vi "BufferWork.vi"(8 "SizeOfArray":i32, 11 "InputArray":i32[](array[numeric])) -> (0 "Index":i32, 3 "OutputArray":i32[](array[numeric]))   [LabVIEW 2020]
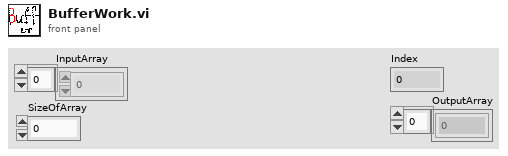
[diagram p1: front panel]
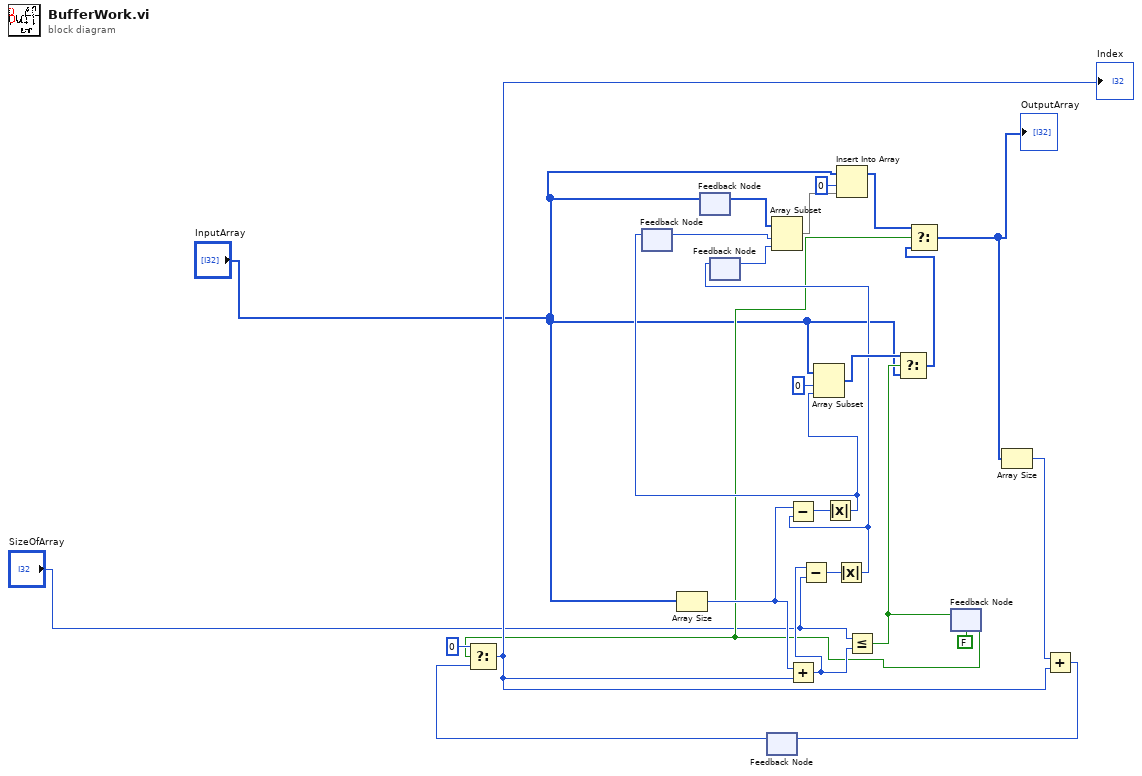
[diagram p0: block diagram]
diagram:
  n1 = feedback #1() -> (w14:i32)  [unwired: 1 in]
  n2 = Array Size(array="InputArray") -> (size(s)=w8:i32)
  n3 = feedback #2() -> (w15:i32[])  [unwired: 1 in]
  n4 = feedback-in #2("InputArray") -> ()
  n5 = feedback #3() -> (w12:i32)  [unwired: 1 in]
  n6 = feedback #4() -> (w4:i32)  [unwired: 1 in]
  n7 = Array Subset(array=w15, index=w14, length=w12) -> (w22:i32[])
  n8 = Insert Into Array(array="InputArray", index=0, new element=w22) -> (w20:i32[])
  n9 = feedback #5(FALSE) -> (w3:bool)
  n10 = Select(t=0, s=w3, f=w4) -> (s? t:f=w6:i32)
  "Index" <- w6
  n11 = Add(x=w8, y=w6) -> (x+y=w9:i32)
  n12 = Subtract(x=w9, y="SizeOfArray") -> (x-y=w16:i32)
  n13 = Absolute Value(x=w16) -> (abs(x)=w13:i32)
  n14 = feedback-in #3(w13) -> ()
  n15 = Subtract(x=w8, y=w13) -> (x-y=w17:i32)
  n16 = Absolute Value(x=w17) -> (abs(x)=w11:i32)
  n17 = feedback-in #1(w11) -> ()
  n18 = Array Subset(array="InputArray", index=0, length=w11) -> (w24:i32[])
  n19 = Less Or Equal?(x="SizeOfArray", y=w9) -> (x <= y?=w10:bool)
  n20 = Select(t=w24, s=w10, f="InputArray") -> (s? t:f=w23:i32[])
  n21 = Select(t=w20, s=w3, f=w23) -> (s? t:f=w19:i32[])
  "OutputArray" <- w19
  n22 = feedback-in #5(w10) -> ()
  n23 = Array Size(array=w19) -> (size(s)=w7:i32)
  n24 = Add(x=w7, y=w6) -> (x+y=w5:i32)
  n25 = feedback-in #4(w5) -> ()
